vi "Input_Digital.vi"() -> ()   [LabVIEW 2018]
uses:
  <vilib>/DAQmx/read.llb/DAQmx Read (Digital Wfm 1Chan 1Samp).vi
  <vilib>/DAQmx/create/channels.llb/DAQmx Create Channel (DI-Digital Input).vi
  <vilib>/DAQmx/miscellaneous.llb/DAQmx Fill In Error Info.vi
panel:
  out "디지털 웨이브폼 그래프":digitalwaveform(graph)
  out "data":digitalwaveform(waveform)={"t0"=timestamp(0 s since 1904-01-01), "dt"=0.0, "Y"={"transitions"=[], "data"=[]}, "error"={"status"=FALSE, "code"=37421928, "source"=""}} caption="데이터"
  in  "정지":bool
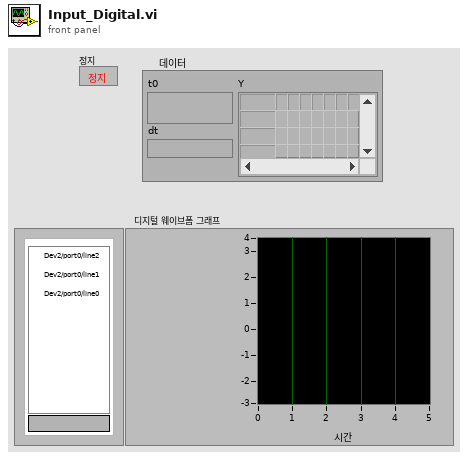
[diagram p1: front panel]
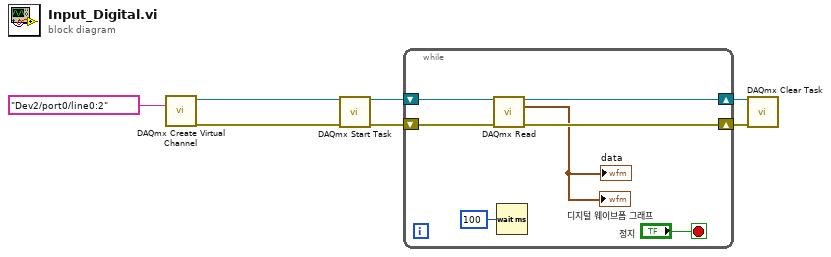
[diagram p0: block diagram]
diagram:
  n1 = call-poly <vilib>:"DAQmx Create Virtual Channel.vi"("lines"=tag "Dev2/port0/line0:2") -> ("task out"=w7:refnum<k21>, "error out"=w6:errorcluster)  [unwired: 13 in]
  n2 = call <vilib>:"DAQmx Start Task.vi"("task/channels in"=w7, "error in"=w6) -> ("task out"=w5:refnum<k21>, "error out"=w4:errorcluster)  [unwired: 12 in]
  n3 = while {
    shift-right: [w12] -> w3
    shift-left: w5 -> [w14]
    shift-right: [w11] -> w2
    shift-left: w4 -> [w13]
    stop <- "정지" stop-if-true
    n4 = call-poly <vilib>:"DAQmx Read.vi"("task/channels in"=w14, "error in"=w13) -> ("task out"=w12:refnum<k21>, "data"=→"data" →"디지털 웨이브폼 그래프":digitalwaveform, "error out"=w11:errorcluster)  [unwired: 11 in]
    n5 = Wait (ms)(milliseconds to wait=u32 100 ("대기 시간 (ms)")) -> ()  [unwired: 1 out]
  }
  n6 = call <vilib>:"DAQmx Clear Task.vi"("task in"=w3, "error in"=w2) -> ()  [unwired: 13 in, 1 out]
